vi "T564_TriggerSourceFromSETresponse.vi"(8 "error in":errorcluster, 11 "String":string) -> (0 "error out":errorcluster, 3 "TriggerSource":T1)   [LabVIEW 2020]
uses:
  TypeDefs/TriggerSource.ctl
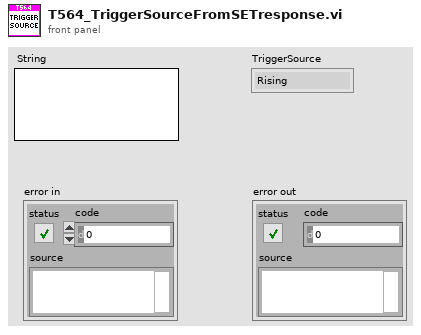
[diagram p1: front panel]
types:
  T1 = typedef "TriggerSource.ctl" = enum16{"Rising", "Falling", "Internal 80MHz", "Internal DDS", "Remote", "Disabled"}
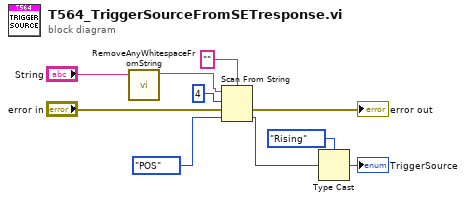
[diagram p0: block diagram]
diagram:
  n1 = call "RemoveAnyWhitespaceFromString.vi"("String in"="String") -> ("String out"=w1:string)  [unwired: 10 in]
  n2 = Scan From String(format string="", input string=w1, initial scan location=u32 4, error in="error in", default 1=enum16{"POS", "NEG", "INT", "SYN", "REMOTE"}."POS") -> (error out=→"error out":errorcluster, output 1=w3:enum16{"POS", "NEG", "INT", "SYN", "REMOTE"})  [unwired: 2 out]
  n3 = Type Cast(type=TriggerSource."Rising" ("TriggerSource 2"), x=w3) -> (*(type *) &x=→"TriggerSource":T1)
